vi "5.0.2_HL_Restriction.vi"(6 "Data in":T1, 8 "error in (no error)":errorcluster, 9 "AllControls In":T2, 10 "?":T3, 11 "Message Queue out":T4) -> (0 "error out":errorcluster, 1 "Flow":string, 2 "Data":T3, 3 "Message Queue Out":T4, 4 "Data out":T1)   [LabVIEW 2017]
uses:
  Depends/AMC/subVIs/TypeDefs/amc_Message Queue.ctl
  Depends/AMC/subVIs/TypeDefs/amc_Message.ctl
  Depends/Tools/Keyed Array/Tools_KeyedArray KeyedArray.ctl
  Ctrls/Data.ctl
  Ctrls/AllControls.ctl
  Ctrls/CSV_Data.ctl
  DIPC 692 Daemon API/typdef/get_parameter.ctl
  DIPC 692 Daemon API/typdef/task_detect_test_point.ctl
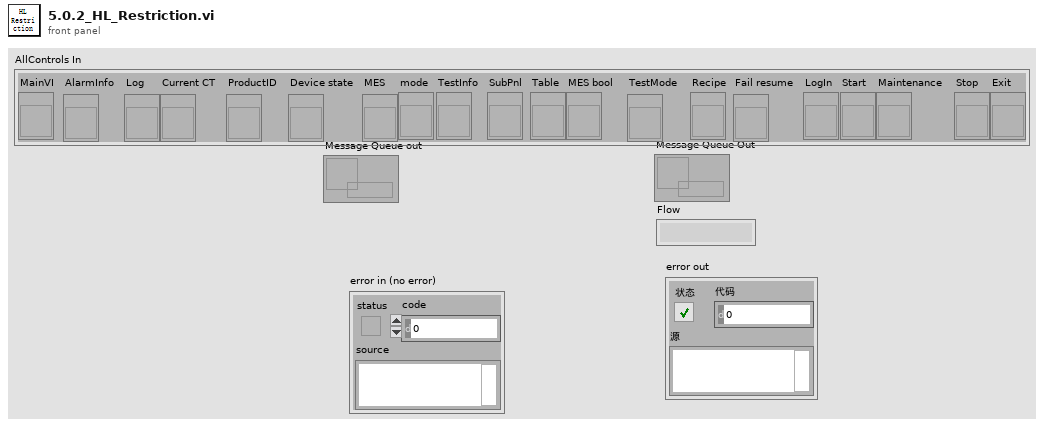
[diagram p1: front panel]
types:
  T1 = typedef "CSV_Data.ctl" = cluster{"Initialisation":cluster{"LMT - Connect UUT (con COM)":string, "LMT - Software Version (rrel)":string, "LMT - Write SKU file (wskuc)":string, "LMT - SKU file name":string, "Connect UUT DDM":string, "Read DDM EOL Timestamp - Mode":string, "Read DDM EOL Timestamp - Timestamp":string, "Read DDM EOL Timestamp - Rig ID":string, "Read DDM EOL Timestamp - Passmark ID":string, "Read DDM EOL Timestamp - Passmark Rev":string, "Software Version before flashing":string, "Read Hardware Serial":string, "UUT DDM SN":string, "Compare DDM SN with MES SN":string, "Backup PCBA Calibration EEPROM Response - CAL":string, "Flash Firmware Version":string, "Check SW Version":string, "Read DDM SW Version after flashing":string, "Set SKU Config":string, "Ready Status":string, "Set Device Mode to EOL":string, "DDM Parameter - Voltage":string, "DDM Parameter - Current":string, "DDM Parameter - Power":string, "DDM Parameter - Speed":string, "DDM Parameter - Pressure":string, "Tester Parameter - Voltage":string, "Tester Parameter - Current":string, "Tester Parameter - Power":string, "Tester Parameter - Ambient Pressure":string, "Tester Parameter - Ambient Temperature":string, "Calculated Parameter - DDM Pressure Corrected":string, "Calculated Parameter - DDM Real Power":string, "Calculated Parameter - Delta V":string}, "BEMF_Calibration":cluster{"Calibration Result - eol_cold_bemf_temp":string, "DDM Ambient Temp":string, "Restriction Plate Diameter":string, "Calibration Result - eol_bemf_mp_cold_coef_a":string, "Calibration Result - eol_bemf_mp_cold_coef_b":string, "Calibration Result - eol_bemf_mp_cold_coef_c":string, "Calibration Result - eol_bemf_lsi_cold_ref_coeffs":string, "Get - Calibration Result - eol_bemf_lsi_speed":string, "Get - Calibration Result - eol_bemf_lsi_integral_0":string, "Calibration Result - eol_bemf_lsi_integral_1":string, "Get - Calibration Result - eol_bemf_lsi_integral_2":string, "Get - Calibration Result - eol_cold_bemf":string, "Get - Calibration Result - eol_cold_bemf_fisf":string, "Finalise Calibration":string, "Compare -Calibration Result - eol_cold_bemf":string, "Compare -Calibration Result - eol_cold_bemf_fisf":string}, "ECO":cluster{"Reset Power Tune":string, "Reset BEMF FISF Calibration":string, "Restriction Plate Diameter":string, "ECO - Stabilisation Time":string, "ECO - DDM Parameter - Voltage":string, "ECO - DDM Parameter - Current":string, "ECO - DDM Parameter - Power":string, "ECO - DDM Parameter - Measured Power":string, "ECO - DDM Parameter - Speed":string, "ECO - DDM Parameter - Pressure":string, "ECO - Tester Parameter - Voltage":string, "ECO - Tester Parameter - Current":string, "ECO - Tester Parameter - Power":string, "ECO - Tester Parameter - Ambient Pressure":string, "ECO - Tester Parameter - Ambient Temperature":string, "ECO - Tester Parameter - Ambient Humidity":string, "ECO - Calculated Parameter - DDM Pressure Corrected":string, "ECO - Calculated Parameter - DDM Real Power":string, "ECO - Calculated Parameter - Delta V":string, "ECO - Calculated Parameter - Flowrate":string, "ECO - Calculated Parameter - Airwatt":string, "ECO - Formula":string, "PT ECO - Power Tune Mode Status":string}, "BOOST":cluster{"Restriction Plate Diameter":string, "BOOST - Stabilisation Time":string, "BOOST - DDM Parameter - Voltage":string, "BOOST - DDM Parameter - Current":string, "BOOST - DDM Parameter - Power":string, "BOOST - DDM Parameter - Measured Power":string, "BOOST - DDM Parameter - Speed":string, "BOOST - DDM Parameter - Pressure":string, "BOOST - Tester Parameter - Voltage":string, "BOOST - Tester Parameter - Current":string, "BOOST - Tester Parameter - Power":string, "BOOST - Tester Parameter - Ambient Pressure":string, "BOOST - Tester Parameter - Ambient Temperature":string, "BOOST - Tester Parameter - Ambient Humidity":string, "BOOST - Calculated Parameter - DDM Pressure Corrected":string, "BOOST - Calculated Parameter - DDM Real Power":string, "BOOST - Calculated Parameter - Delta V":string, "BOOST - Calculated Parameter - Flowrate":string, "BOOST - Calculated Parameter - Airwatt":string, "BOOST - Get AM Presence":string, "Air Muscle Turn Off Status":string, "BOOST - Air Muscle Calculated Parameter - Airwatt B":string, "BOOST - Air Muscle Calculate Airwatt Delta":string, "PT BOOST - Power Tune Mode Status":string, "Finalise Calibration":string, "ECO - Get AW Calibration value":string, "BOOST - Get AW Calibration value":string}, "MAX":cluster{"Restriction Plate Diameter":string, "MAX - Stabilisation Time":string, "Get Average Delta Tmag (LSIdelta_FISFdelta_LSItmag_FISFtmag_IIRtmag)":string, "Get Average Delta Tmag FISF":string, "MAX - DDM Parameter - Voltage":string, "MAX - DDM Parameter - Current":string, "MAX - DDM Parameter - Power":string, "MAX - DDM Parameter - Measured Power":string, "MAX - DDM Parameter - Speed":string, "MAX - DDM Parameter - Pressure":string, "MAX - Tester Parameter - Voltage":string, "MAX - Tester Parameter - Current":string, "MAX - Tester Parameter - Power":string, "MAX - Tester Parameter - Ambient Pressure":string, "MAX - Tester Parameter - Ambient Temperature":string, "MAX - Tester Parameter - Ambient Humidity":string, "MAX - Calculated Parameter - DDM Pressure Corrected":string, "MAX - Calculated Parameter - DDM Real Power":string, "MAX - Calculated Parameter - Delta V":string, "MAX - Calculated Parameter - Flowrate":string, "MAX - Calculated Parameter - Airwatt":string, "MAX_FISF_Check_Average_Delta_Tmag":string, "MAX - FISF - BEMF Finetune Result":string, "MAX tune - Delta P1":string, "MAX tune - Calculated Parameter - Airwatt":string, "Calculate Delta Airwatts - MAX finetune - Delta P2":string, "MAX finetune - DDM Parameter - Voltage":string, "MAX finetune - DDM Parameter - Current":string, "MAX finetune - DDM Parameter - Power":string, "MAX finetune - DDM Parameter - Measured Power":string, "MAX finetune - DDM Parameter - Speed":string, "MAX finetune - DDM Parameter - Pressure":string, "MAX finetune - Tester Parameter - Voltage":string, "MAX finetune - Tester Parameter - Current":string, "MAX finetune - Tester Parameter - Power":string, "MAX finetune - Tester Parameter - Ambient Pressure":string, "MAX finetune - Tester Parameter - Ambient Temperature":string, "MAX finetune - Tester Parameter - Ambient Humidity":string, "MAX finetune - Calculated Parameter - DDM Pressure Corrected":string, "MAX finetune - Calculated Parameter - DDM Real Power":string, "MAX finetune - Calculated Parameter - Delta V":string, "MAX finetune - Calculated Parameter - Flowrate":string, "MAX finetune - Calculated Parameter - Airwatt":string, "Check Derate Result":string, "Delta Tmag FISF":string, "Get Hot BEMF Result":string, "Calculate delta Pressure":string, "Finalise Calibration":string, "Calculate & Check Delta BEMF":string, "Delta P Airwatts Value":string}, "LL":cluster{"DDM Ambient Temp":string, "Restriction Plate Diameter":string, "LL - DDM Parameter - Voltage":string, "LL - DDM Parameter - Current":string, "LL - DDM Parameter - Power":string, "LL - DDM Parameter - Measured Power":string, "LL - DDM Parameter - Speed":string, "LL - DDM Parameter - Pressure":string, "LL - Tester Parameter - Voltage":string, "LL - Tester Parameter - Current":string, "LL - Tester Parameter - Power":string, "LL - DDM Real Power":string, "LL - Calibrate Task Detect LL":string}, "HL":cluster{"HL - DDM Parameter - Voltage":string, "HL - DDM Parameter - Current":string, "HL - DDM Parameter - Power":string, "HL - DDM Parameter - Measured Power":string, "HL - DDM Parameter - Speed":string, "HL - DDM Parameter - Pressure":string, "HL - Tester Parameter - Voltage":string, "HL - Tester Parameter - Current":string, "HL - Tester Parameter - Power":string, "HL - DDM Real Power":string, "HL - Calibrate Task Detect HL":string}, "LH":cluster{"Restriction Plate Diameter":string, "LH - DDM Parameter - Voltage":string, "LH - DDM Parameter - Current":string, "LH - DDM Parameter - Power":string, "LH - DDM Parameter - Measured Power":string, "LH - DDM Parameter - Speed":string, "LH - DDM Parameter - Pressure":string, "LH - Tester Parameter - Voltage":string, "LH - Tester Parameter - Current":string, "LH - Tester Parameter - Power":string, "LH - DDM Real Power":string, "LH - Calibrate Task Detect LH":string}, "HH":cluster{"HH - DDM Parameter - Voltage":string, "HH - DDM Parameter - Current":string, "HH - DDM Parameter - Power":string, "HH - DDM Parameter - Measured Power":string, "HH - DDM Parameter - Speed":string, "HH - DDM Parameter - Pressure":string, "HH - Tester Parameter - Voltage":string, "HH - Tester Parameter - Current":string, "HH - Tester Parameter - Power":string, "HH - DDM Real Power":string, "HH - Calibrate Task Detect HH":string}, "Inlet Blockage Calibration":cluster{"Inlet Blockage Calibration - DDM Parameter - Voltage":string, "Inlet Blockage Calibration - DDM Parameter - Current":string, "Inlet Blockage Calibration - DDM Parameter - Power":string, "Inlet Blockage Calibration - DDM Parameter - Measured Power":string, "Inlet Blockage Calibration - DDM Parameter - Speed":string, "Inlet Blockage Calibration - DDM Parameter - Pressure":string, "Inlet Blockage Calibration - Tester Parameter - Voltage":string, "Inlet Blockage Calibration - Tester Parameter - Current":string, "Inlet Blockage Calibration - Tester Parameter - Power":string, "Inlet Blockage Calibration - DDM Real Power":string, "Calibration Inlet Blockage_E":string, "Finalise Calibration":string, "Get Task Detect LL":string, "Get Task Detect HL":string, "Get Task Detect LH":string, "Get Task Detect HH":string, "Calibration Inlet Blockage":string, "Calibration eol cold bemf temp":string}, "GOOD":cluster{"GOOD UNIT - Clear EEPROM Error Log":string, "GOOD UNIT - Write Product Timestamp - Mode":string, "GOOD UNIT - Write Product Timestamp - Timestamp":string, "GOOD UNIT - Write Product Timestamp - Rig ID":string, "GOOD UNIT - Write Product Timestamp - Passmark ID":string, "GOOD UNIT - Write Product Timestamp - Passmark Rev":string, "GOOD UNIT - Set Device Mode to PROD":string, "GOOD UNIT - Backup PCBA Calibration EEPROM Response":string, "GOOD UNIT - Check Security Bit":string, "GOOD UNIT - Set Calibration Lock":string, "GOOD UNIT - Get_Calibration_Lock":string, "GOOD UNIT - Disconnect UUT":string}, "NG":cluster{"NG UNIT - Read NVM Error":string, "NG UNIT - Set Device Mode to FCT":string, "NG UNIT - Backup PCBA Calibration EEPROM Response - CAL":string, "NG UNIT - Backup PCBA Calibration EEPROM Response - ERROR":string, "NG UNIT - Backup PCBA Calibration EEPROM Response - USAGE":string, "NG UNIT - Disconnect UUT":string}, "SN":string, "Table":string[][], "Count":cluster{"Total":i32, "OK":i32, "NG":i32, "Yield":dbl}, "Start Time":timestamp, "daemon reference":refnum<k5>, "CT":dbl, "Config":string[][], "OK/NG":bool, "Station ID":string, "MES DDM SN":string, "MES PCBA SN":string, "Retest":string, "UID":string, "Initialisation_Status":cluster{"LMT - Connect UUT (con COM)":string, "LMT - Software Version (rrel)":string, "LMT - Write SKU file (wskuc)":string, "LMT - SKU file name":string, "Connect UUT DDM":string, "Read DDM EOL Timestamp - Mode":string, "Read DDM EOL Timestamp - Timestamp":string, "Read DDM EOL Timestamp - Rig ID":string, "Read DDM EOL Timestamp - Passmark ID":string, "Read DDM EOL Timestamp - Passmark Rev":string, "Software Version before flashing":string, "Read Hardware Serial":string, "UUT DDM SN":string, "Compare DDM SN with MES SN":string, "Backup PCBA Calibration EEPROM Response - CAL":string, "Flash Firmware Version":string, "Check SW Version":string, "Read DDM SW Version after flashing":string, "Set SKU Config":string, "Ready Status":string, "Set Device Mode to EOL":string, "DDM Parameter - Voltage":string, "DDM Parameter - Current":string, "DDM Parameter - Power":string, "DDM Parameter - Speed":string, "DDM Parameter - Pressure":string, "Tester Parameter - Voltage":string, "Tester Parameter - Current":string, "Tester Parameter - Power":string, "Tester Parameter - Ambient Pressure":string, "Tester Parameter - Ambient Temperature":string, "Calculated Parameter - DDM Pressure Corrected":string, "Calculated Parameter - DDM Real Power":string, "Calculated Parameter - Delta V":string}, "BEMF_Calibration_Status":cluster{"Calibration Result - eol_cold_bemf_temp":string, "DDM Ambient Temp":string, "Restriction Plate Diameter":string, "Calibration Result - eol_bemf_mp_cold_coef_a":string, "Calibration Result - eol_bemf_mp_cold_coef_b":string, "Calibration Result - eol_bemf_mp_cold_coef_c":string, "Calibration Result - eol_bemf_lsi_cold_ref_coeffs":string, "Get - Calibration Result - eol_bemf_lsi_speed":string, "Get - Calibration Result - eol_bemf_lsi_integral_0":string, "Calibration Result - eol_bemf_lsi_integral_1":string, "Get - Calibration Result - eol_bemf_lsi_integral_2":string, "Get - Calibration Result - eol_cold_bemf":string, "Get - Calibration Result - eol_cold_bemf_fisf":string, "Finalise Calibration":string, "Compare -Calibration Result - eol_cold_bemf":string, "Compare -Calibration Result - eol_cold_bemf_fisf":string}, "ECO_Status":cluster{"Reset Power Tune":string, "Reset BEMF FISF Calibration":string, "Restriction Plate Diameter":string, "ECO - Stabilisation Time":string, "ECO - DDM Parameter - Voltage":string, "ECO - DDM Parameter - Current":string, "ECO - DDM Parameter - Power":string, "ECO - DDM Parameter - Measured Power":string, "ECO - DDM Parameter - Speed":string, "ECO - DDM Parameter - Pressure":string, "ECO - Tester Parameter - Voltage":string, "ECO - Tester Parameter - Current":string, "ECO - Tester Parameter - Power":string, "ECO - Tester Parameter - Ambient Pressure":string, "ECO - Tester Parameter - Ambient Temperature":string, "ECO - Tester Parameter - Ambient Humidity":string, "ECO - Calculated Parameter - DDM Pressure Corrected":string, "ECO - Calculated Parameter - DDM Real Power":string, "ECO - Calculated Parameter - Delta V":string, "ECO - Calculated Parameter - Flowrate":string, "ECO - Calculated Parameter - Airwatt":string, "ECO - Formula":string, "PT ECO - Power Tune Mode Status":string}, "BOOST_Status":cluster{"Restriction Plate Diameter":string, "BOOST - Stabilisation Time":string, "BOOST - DDM Parameter - Voltage":string, "BOOST - DDM Parameter - Current":string, "BOOST - DDM Parameter - Power":string, "BOOST - DDM Parameter - Measured Power":string, "BOOST - DDM Parameter - Speed":string, "BOOST - DDM Parameter - Pressure":string, "BOOST - Tester Parameter - Voltage":string, "BOOST - Tester Parameter - Current":string, "BOOST - Tester Parameter - Power":string, "BOOST - Tester Parameter - Ambient Pressure":string, "BOOST - Tester Parameter - Ambient Temperature":string, "BOOST - Tester Parameter - Ambient Humidity":string, "BOOST - Calculated Parameter - DDM Pressure Corrected":string, "BOOST - Calculated Parameter - DDM Real Power":string, "BOOST - Calculated Parameter - Delta V":string, "BOOST - Calculated Parameter - Flowrate":string, "BOOST - Calculated Parameter - Airwatt":string, "BOOST - Get AM Presence":string, "Air Muscle Turn Off Status":string, "BOOST - Air Muscle Calculated Parameter - Airwatt B":string, "BOOST - Air Muscle Calculate Airwatt Delta":string, "PT BOOST - Power Tune Mode Status":string, "Finalise Calibration":string, "ECO - Get AW Calibration value":string, "BOOST - Get AW Calibration value":string}, "MAX_Status":cluster{"Restriction Plate Diameter":string, "MAX - Stabilisation Time":string, "Get Average Delta Tmag (LSIdelta_FISFdelta_LSItmag_FISFtmag_IIRtmag)":string, "Get Average Delta Tmag FISF":string, "MAX - DDM Parameter - Voltage":string, "MAX - DDM Parameter - Current":string, "MAX - DDM Parameter - Power":string, "MAX - DDM Parameter - Measured Power":string, "MAX - DDM Parameter - Speed":string, "MAX - DDM Parameter - Pressure":string, "MAX - Tester Parameter - Voltage":string, "MAX - Tester Parameter - Current":string, "MAX - Tester Parameter - Power":string, "MAX - Tester Parameter - Ambient Pressure":string, "MAX - Tester Parameter - Ambient Temperature":string, "MAX - Tester Parameter - Ambient Humidity":string, "MAX - Calculated Parameter - DDM Pressure Corrected":string, "MAX - Calculated Parameter - DDM Real Power":string, "MAX - Calculated Parameter - Delta V":string, "MAX - Calculated Parameter - Flowrate":string, "MAX - Calculated Parameter - Airwatt":string, "MAX_FISF_Check_Average_Delta_Tmag":string, "MAX - FISF - BEMF Finetune Result":string, "MAX tune - Delta P1":string, "MAX tune - Calculated Parameter - Airwatt":string, "Calculate Delta Airwatts - MAX finetune - Delta P2":string, "MAX finetune - DDM Parameter - Voltage":string, "MAX finetune - DDM Parameter - Current":string, "MAX finetune - DDM Parameter - Power":string, "MAX finetune - DDM Parameter - Measured Power":string, "MAX finetune - DDM Parameter - Speed":string, "MAX finetune - DDM Parameter - Pressure":string, "MAX finetune - Tester Parameter - Voltage":string, "MAX finetune - Tester Parameter - Current":string, "MAX finetune - Tester Parameter - Power":string, "MAX finetune - Tester Parameter - Ambient Pressure":string, "MAX finetune - Tester Parameter - Ambient Temperature":string, "MAX finetune - Tester Parameter - Ambient Humidity":string, "MAX finetune - Calculated Parameter - DDM Pressure Corrected":string, "MAX finetune - Calculated Parameter - DDM Real Power":string, "MAX finetune - Calculated Parameter - Delta V":string, "MAX finetune - Calculated Parameter - Flowrate":string, "MAX finetune - Calculated Parameter - Airwatt":string, "Check Derate Result":string, "Delta Tmag FISF":string, "Get Hot BEMF Result":string, "Calculate delta Pressure":string, "Finalise Calibration":string, "Calculate & Check Delta BEMF":string, "Delta P Airwatts Value":string}, "LL_Status":cluster{"DDM Ambient Temp":string, "Restriction Plate Diameter":string, "LL - DDM Parameter - Voltage":string, "LL - DDM Parameter - Current":string, "LL - DDM Parameter - Power":string, "LL - DDM Parameter - Measured Power":string, "LL - DDM Parameter - Speed":string, "LL - DDM Parameter - Pressure":string, "LL - Tester Parameter - Voltage":string, "LL - Tester Parameter - Current":string, "LL - Tester Parameter - Power":string, "LL - DDM Real Power":string, "LL - Calibrate Task Detect LL":string}, "HL_Status":cluster{"HL - DDM Parameter - Voltage":string, "HL - DDM Parameter - Current":string, "HL - DDM Parameter - Power":string, "HL - DDM Parameter - Measured Power":string, "HL - DDM Parameter - Speed":string, "HL - DDM Parameter - Pressure":string, "HL - Tester Parameter - Voltage":string, "HL - Tester Parameter - Current":string, "HL - Tester Parameter - Power":string, "HL - DDM Real Power":string, "HL - Calibrate Task Detect HL":string}, "LH_Status":cluster{"Restriction Plate Diameter":string, "LH - DDM Parameter - Voltage":string, "LH - DDM Parameter - Current":string, "LH - DDM Parameter - Power":string, "LH - DDM Parameter - Measured Power":string, "LH - DDM Parameter - Speed":string, "LH - DDM Parameter - Pressure":string, "LH - Tester Parameter - Voltage":string, "LH - Tester Parameter - Current":string, "LH - Tester Parameter - Power":string, "LH - DDM Real Power":string, "LH - Calibrate Task Detect LH":string}, "HH_Status":cluster{"HH - DDM Parameter - Voltage":string, "HH - DDM Parameter - Current":string, "HH - DDM Parameter - Power":string, "HH - DDM Parameter - Measured Power":string, "HH - DDM Parameter - Speed":string, "HH - DDM Parameter - Pressure":string, "HH - Tester Parameter - Voltage":string, "HH - Tester Parameter - Current":string, "HH - Tester Parameter - Power":string, "HH - DDM Real Power":string, "HH - Calibrate Task Detect HH":string}, "Inlet Blockage Calibration_Status":cluster{"Inlet Blockage Calibration - DDM Parameter - Voltage":string, "Inlet Blockage Calibration - DDM Parameter - Current":string, "Inlet Blockage Calibration - DDM Parameter - Power":string, "Inlet Blockage Calibration - DDM Parameter - Measured Power":string, "Inlet Blockage Calibration - DDM Parameter - Speed":string, "Inlet Blockage Calibration - DDM Parameter - Pressure":string, "Inlet Blockage Calibration - Tester Parameter - Voltage":string, "Inlet Blockage Calibration - Tester Parameter - Current":string, "Inlet Blockage Calibration - Tester Parameter - Power":string, "Inlet Blockage Calibration - DDM Real Power":string, "Calibration Inlet Blockage_E":string, "Finalise Calibration":string, "Get Task Detect LL":string, "Get Task Detect HL":string, "Get Task Detect LH":string, "Get Task Detect HH":string, "Calibration Inlet Blockage":string, "Calibration eol cold bemf temp":string}, "GOOD_Status":cluster{"GOOD UNIT - Clear EEPROM Error Log":string, "GOOD UNIT - Write Product Timestamp - Mode":string, "GOOD UNIT - Write Product Timestamp - Timestamp":string, "GOOD UNIT - Write Product Timestamp - Rig ID":string, "GOOD UNIT - Write Product Timestamp - Passmark ID":string, "GOOD UNIT - Write Product Timestamp - Passmark Rev":string, "GOOD UNIT - Set Device Mode to PROD":string, "GOOD UNIT - Backup PCBA Calibration EEPROM Response":string, "GOOD UNIT - Check Security Bit":string, "GOOD UNIT - Set Calibration Lock":string, "GOOD UNIT - Get_Calibration_Lock":string, "GOOD UNIT - Disconnect UUT":string}, "NG_Status":cluster{"NG UNIT - Read NVM Error":string, "NG UNIT - Set Device Mode to FCT":string, "NG UNIT - Backup PCBA Calibration EEPROM Response - CAL":string, "NG UNIT - Backup PCBA Calibration EEPROM Response - ERROR":string, "NG UNIT - Backup PCBA Calibration EEPROM Response - USAGE":string, "NG UNIT - Disconnect UUT":string}, "SKU":string, "Plate_Diameter":string, "Alarm":string}
  T2 = typedef "AllControls.ctl" = cluster{"MainVI":refnum<vi>, "AlarmInfo":refnum<vi>, "Log":refnum<vi>, "Current CT":refnum<vi>, "ProductID":refnum<vi>, "Device state":refnum<vi>, "MES":refnum<vi>, "mode":refnum<vi>, "TestInfo":refnum<vi>, "SubPnl":refnum<vi>, "Table":refnum<vi>, "MES bool":refnum<vi>, "TestMode":refnum<vi>, "Recipe":refnum<vi>, "Fail resume":refnum<vi>, "LogIn":refnum<vi>, "Start":refnum<vi>, "Maintenance":refnum<vi>, "Stop":refnum<vi>, "Exit":refnum<vi>}
  T3 = typedef "Data.ctl" = cluster{"Initialisation":cluster{"DDM_Parameter":dbl[], "DDM_Parameter_status":bool[], "Get_Tester_Parameter":dbl[], "Get_Tester_Parameter_status":bool[], "Cal_Tester_Parameter":dbl[], "Cal_Tester_Parameter_status":bool[], "sw_version_before_status":bool, "sw_version_after_status":bool, "Set_SKU_Config_With_LMT_status":bool, "FCT_timestamp_status":bool, "LMT_Connect_to_UUT_status":bool}, "BEMF_Calibration":cluster{"Read_ambient_temperature":dbl, "Calibration_Vaule":dbl[], "Calibration_Vaule _B":dbl[], "Calibration_Vaule_status":bool[], "Calibration_Vaule_B_status":bool[]}, "ECO":cluster{"DDM_Parameter":dbl[], "DDM_Parameter_status":bool[], "Get_Tester_Parameter":dbl[], "Get_Tester_Parameter_status":bool[], "Cal_Tester_Parameter":dbl[], "Cal_Tester_Parameter_status":bool[], "DDM_Parameter_after_power_tune":dbl[], "Get_Tester_Parameter_after_power_tune":dbl[], "Cal_Tester_Parameter_after_power_tune":dbl[], "Cal_Tester_Parameter_after_power_tune_status":bool[], "Delta_P":dbl}, "BOOST":cluster{"DDM_Parameter":dbl[], "DDM_Parameter_status":bool[], "Get_Tester_Parameter":dbl[], "Get_Tester_Parameter_status":bool[], "Cal_Tester_Parameter":dbl[], "Cal_Tester_Parameter_status":bool[], "DDM_Parameter_after_power_tune":dbl[], "Get_Tester_Parameter_after_power_tune":dbl[], "Cal_Tester_Parameter_after_power_tune":dbl[], "Cal_Tester_Parameter_after_power_tune_status":bool[], "airwatts_am_off":dbl, "AW_Delta_(AM_on_and_off)":dbl, "AW_Delta_(AM_on_and_off)_Status":bool, "Delta_P":dbl}, "MAX":cluster{"Average_Tmag_Data":cluster{"LSI Delta in degC":dbl, "FISF Delta in degc":dbl, "LSI Tmag in degC":dbl, "Fisf Tmag in degC":dbl, "IIR Tmag in degC":dbl}, "DDM_Parameter":dbl[], "DDM_Parameter_status":bool[], "Get_Tester_Parameter":dbl[], "Get_Tester_Parameter_status":bool[], "Cal_Tester_Parameter":dbl[], "BEMF_Finetune":cluster{"eol_bemf_mp_cold_coef_c":dbl, "eol_cold_bemf_fisf_offset":dbl}, "AW_Tune":cluster{"delta_P1":dbl, "delta_P_Setting":dbl}, "DDM_Parameter_after_Airwatts_Tune":dbl[], "Get_Tester_Parameter_after_Airwatts_Tune":dbl[], "Cal_Tester_Parameter_after_Airwatts_Tune":dbl[], "DDM_Parameter_after_Airwatts_Finetune":dbl[], "Get_Tester_Parameter_after_Airwatts_Finetune":dbl[], "Cal_Tester_Parameter_after_Airwatts_Finetune":dbl[], "AW_Finetune":cluster{"delta_P2":dbl, "delta_P_Setting":dbl}, "Delta_Tmag_after_tune":cluster{"LSI Delta in degC":dbl, "FISF Delta in degc":dbl, "LSI Tmag in degC":dbl, "Fisf Tmag in degC":dbl, "IIR Tmag in degC":dbl}, "Hot Bemf in mV":dbl, "DDM_Pressure":dbl, "Delta_Pressure":dbl, " Cold Bemf in mV":dbl, " delta Bemf":dbl, " delta p":dbl, "Delta_Pressure_status":bool, " delta Bemf_status":bool, "LSI Delta in degC_status":bool, "FISF Delta in degc_status":bool, "Max_check_derate_status_status":bool, "Average_All_data":dbl[][], "Average_Tmag_Data_status":bool[], "Average_Tmag_Data_after_tune_status":bool[], "Cal_Tester_Parameter_status":bool[], "Cal_Tester_Parameter_status_after_Airwatts_Tune":bool[], "Cal_Tester_Parameter_status_after_Airwatts_FineTune":bool[]}, "Task_Detect_Calib":cluster{"LL":cluster{"DDM_Parameter":dbl[], "DDM_Parameter_status":bool[], "Get_Tester_Parameter":dbl[], "Get_Tester_Parameter_status":bool[], "Set_task_detect_A":dbl, "Set_task_detect_A_Status":bool}, "HL":cluster{"DDM_Parameter":dbl[], "DDM_Parameter_status":bool[], "Get_Tester_Parameter":dbl[], "Get_Tester_Parameter_status":bool[], "Set_task_detect_B":dbl, "Set_task_detect_B_Status":bool}, "LH":cluster{"DDM_Parameter":dbl[], "DDM_Parameter_status":bool[], "Get_Tester_Parameter":dbl[], "Get_Tester_Parameter_status":bool[], "Set_task_detect_C":dbl, "Set_task_detect_C_Status":bool}, "HH":cluster{"DDM_Parameter":dbl[], "DDM_Parameter_status":bool[], "Get_Tester_Parameter":dbl[], "Get_Tester_Parameter_status":bool[], "Set_task_detect_D":dbl, "Read_and_check_calibration_Status":bool[], "Set_task_detect_D_Status":bool}, "Get_eol_inlet_blockage_E":dbl, "Calib_vaule":cluster{"Get_task_detect_LL":dbl, "Get_task_detect_HL":dbl, "Get_task_detect_LH":dbl, "Get_task_detect_HH":dbl, "eol_inlet_blockage":dbl, "eol_code_bemf_temp":dbl}, "calibrated temp":dbl, "Inlet_Blockage_Calibration":cluster{"DDM_Parameter":dbl[], "DDM_Parameter_status":bool[], "Get_Tester_Parameter":dbl[], "Get_Tester_Parameter_status":bool[]}, "Get_eol_inlet_blockage_E_Status":bool}, "good":cluster{"Write_Product_TS":cluster{"TIMESTAMP":i64, "RIG_ID":i64, "PASSMARK_ID":i64, "PASSMARK_REV":i64}, "Read_Product_TS":cluster{"TIMESTAMP":i64, "RIG_ID":i64, "PASSMARK_ID":i64, "PASSMARK_REV":i64}, "Good_Check_Secuity_Bit_Stauts":bool}}
  T4 = typedef "amc_Message Queue.ctl" = refnum<queue>
  T5 = typedef "HD Config.ctl" = cluster{" PC":cluster{"PC Address":u8[], "PC Port":i32}, "FCO":cluster{"COM":refnum<visa-resource-name>, "Baudrate":u32}, "DC Power ":cluster{"COM":refnum<visa-resource-name>, "Baudrate":u32}, "PW3336":cluster{"COM":refnum<visa-resource-name>, "Baudrate":u32}, "Lefoo":cluster{"COM":refnum<visa-resource-name>, "Baudrate":u32}, "AI Model":cluster{"COM":refnum<visa-resource-name>, "Baudrate":u32}, "DIPC":cluster{"COM":refnum<visa-resource-name>}, "RFID":cluster{"IP Address":string, "Port":u16, "Retry":u16}, "Motor":cluster{"COM":refnum<visa-resource-name>, "Baudrate":u32}, "Fail_resume_mode":bool, "GRR":bool}
  T6 = typedef "get_parameter.ctl" = string
  T7 = typedef "task_detect_test_point.ctl" = enum16{"LL", "HL", "LH", "HH"}
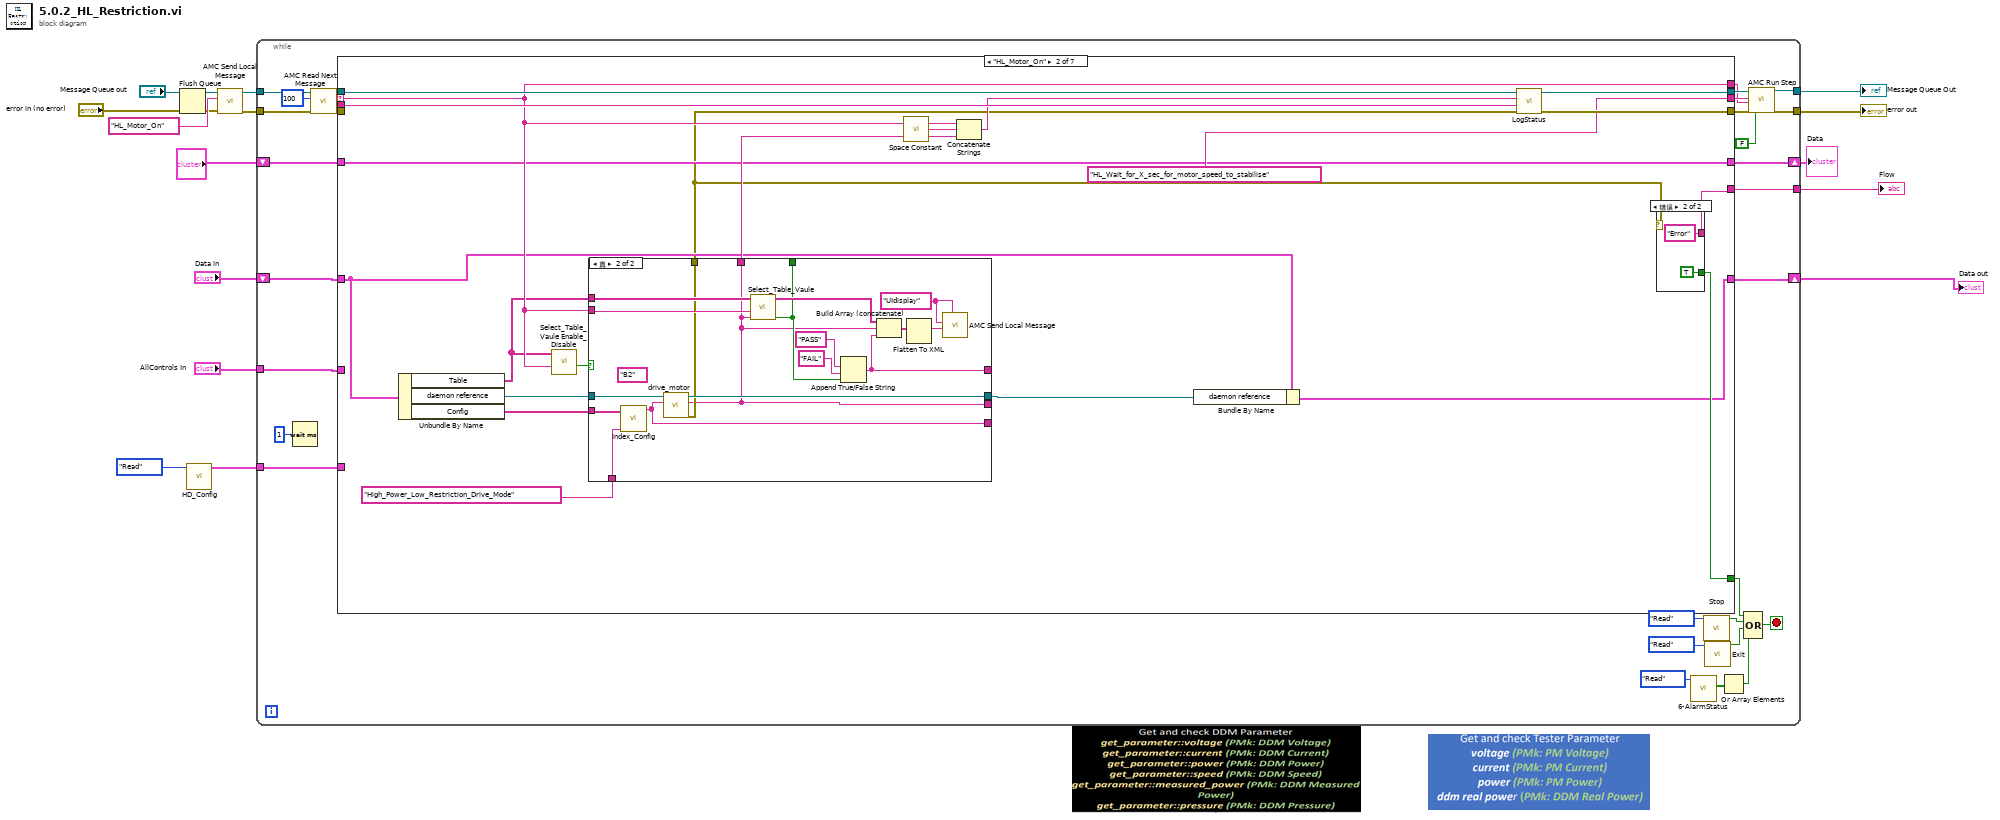
[diagram p0: block diagram]
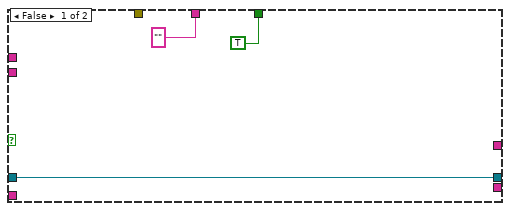
[diagram p4: hidden frame]
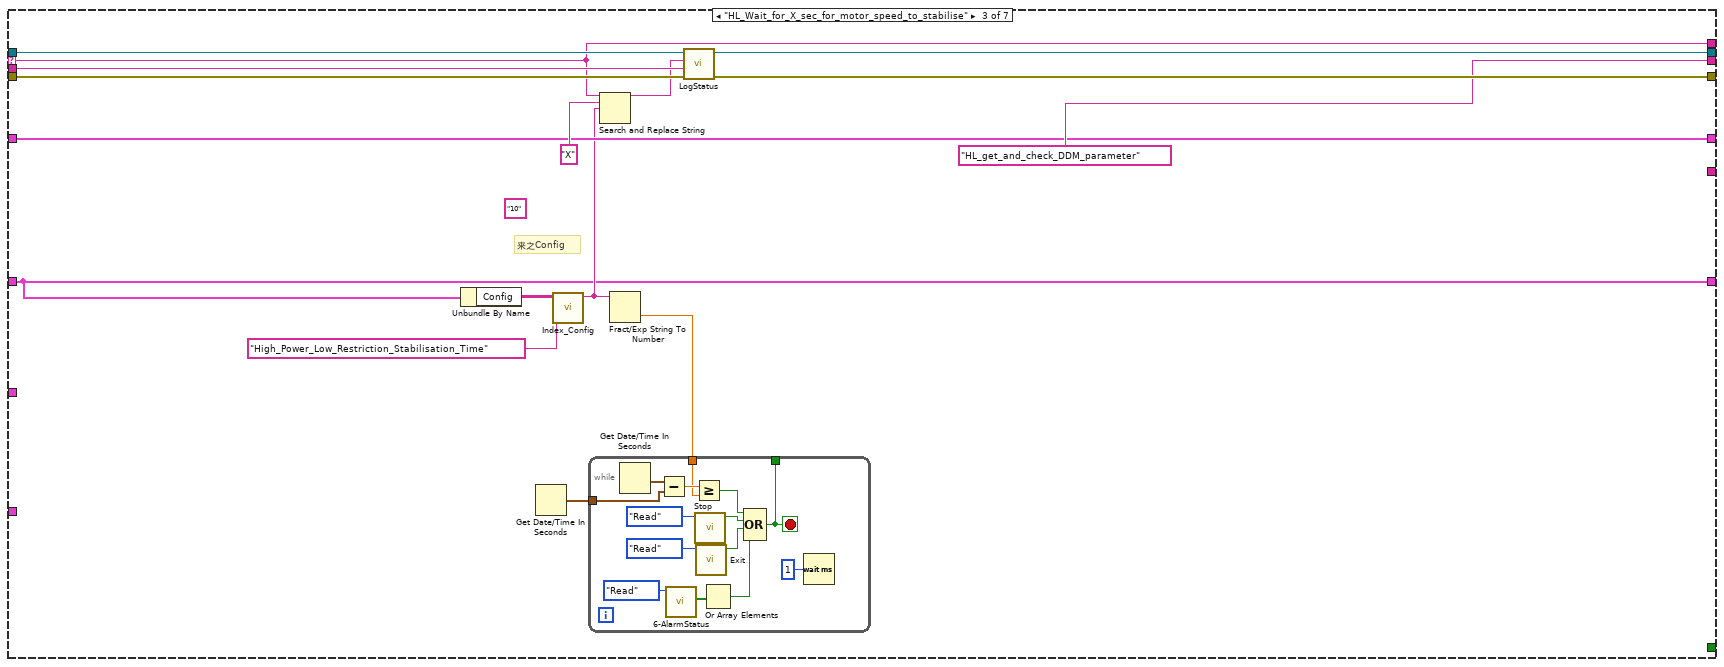
[diagram p5: hidden frame]
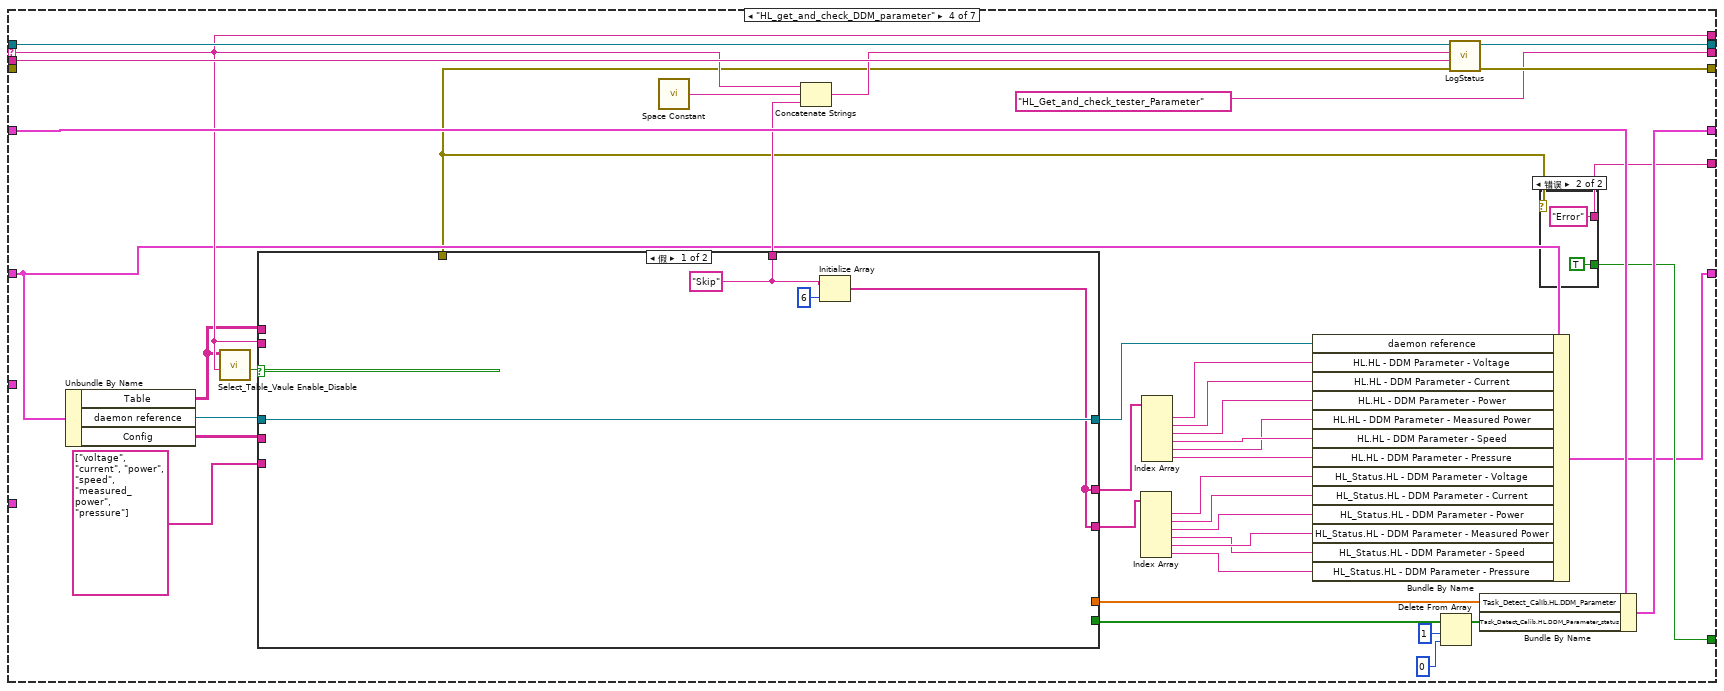
[diagram p6: hidden frame]
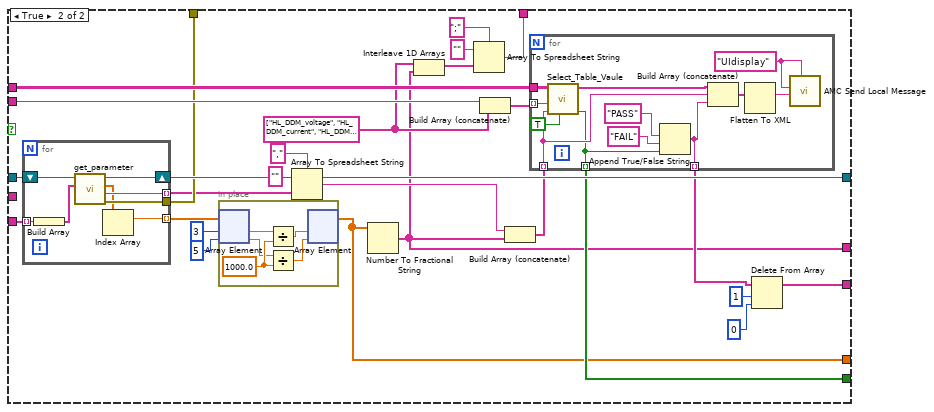
[diagram p8: hidden frame]
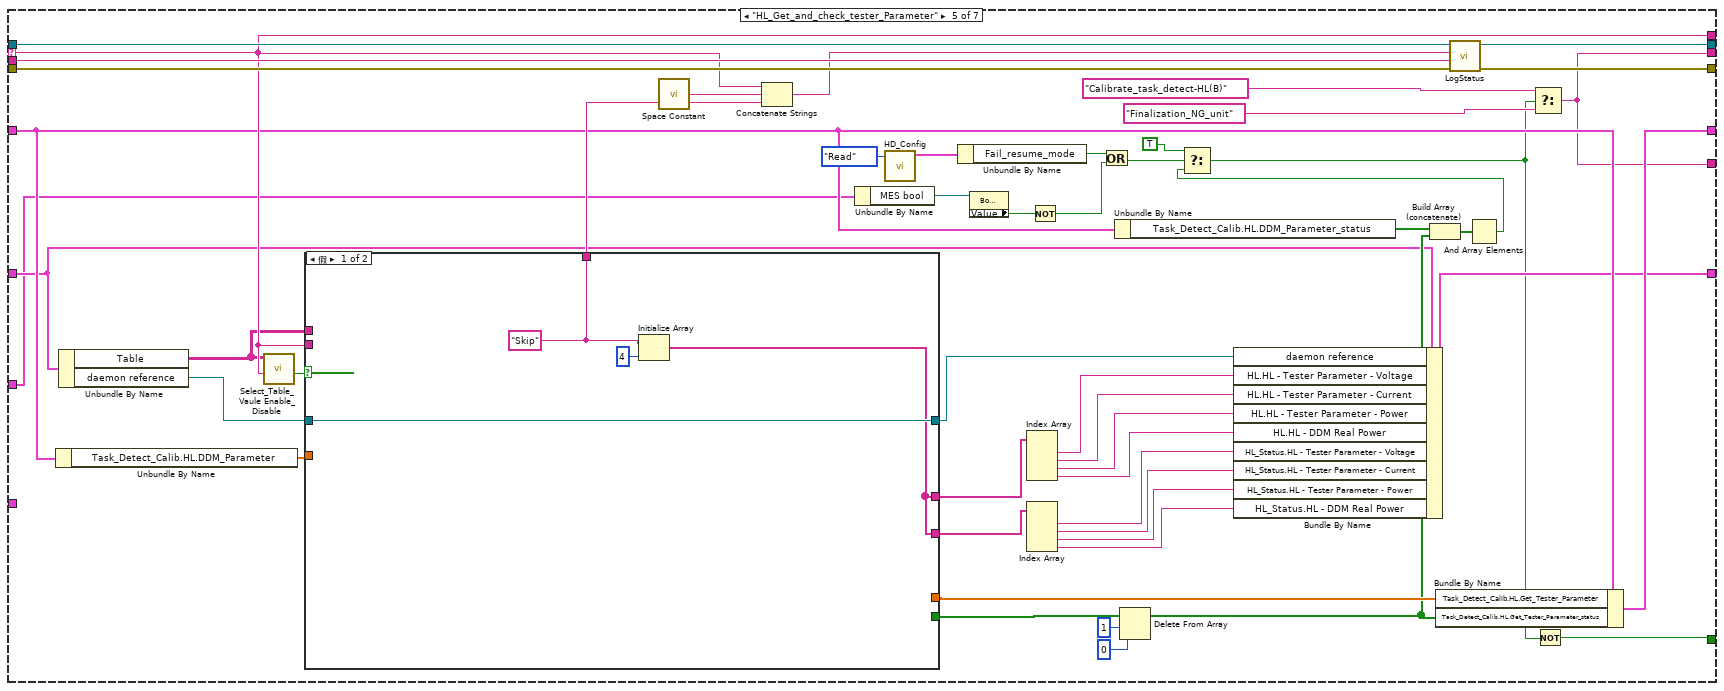
[diagram p9: hidden frame]
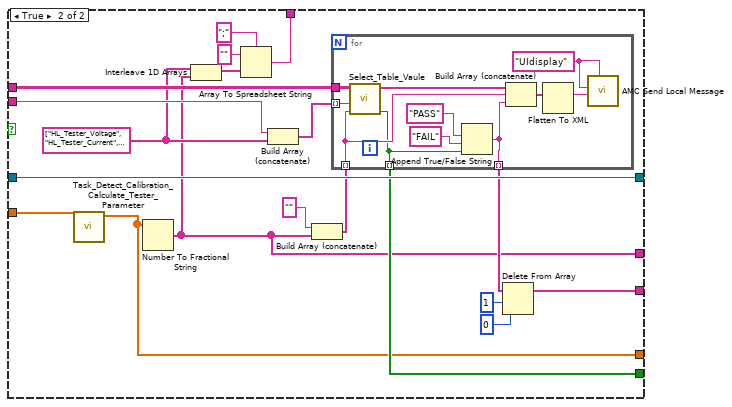
[diagram p10: hidden frame]
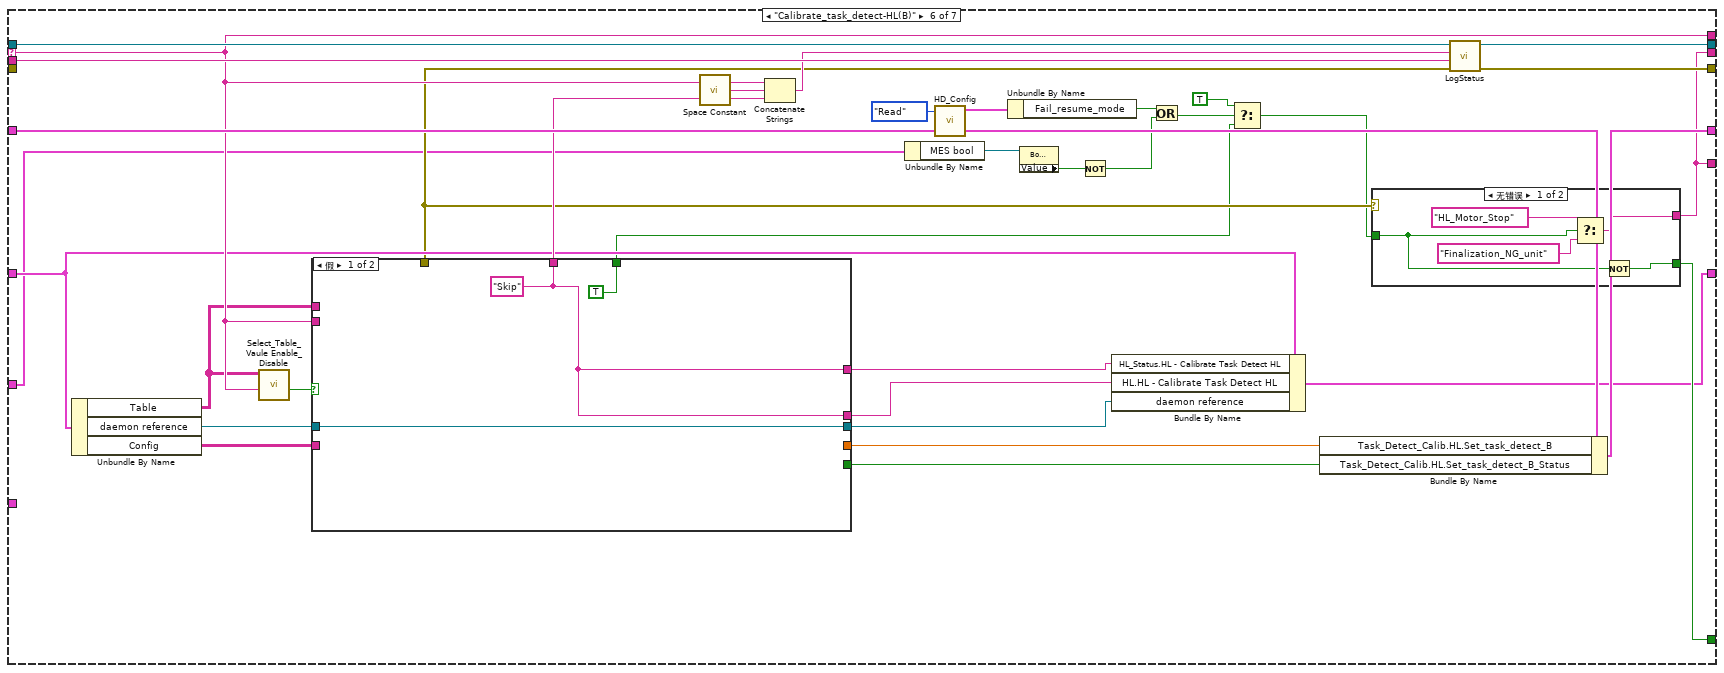
[diagram p11: hidden frame]
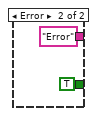
[diagram p12: hidden frame]
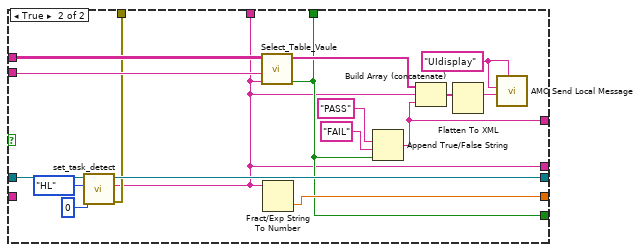
[diagram p13: hidden frame]
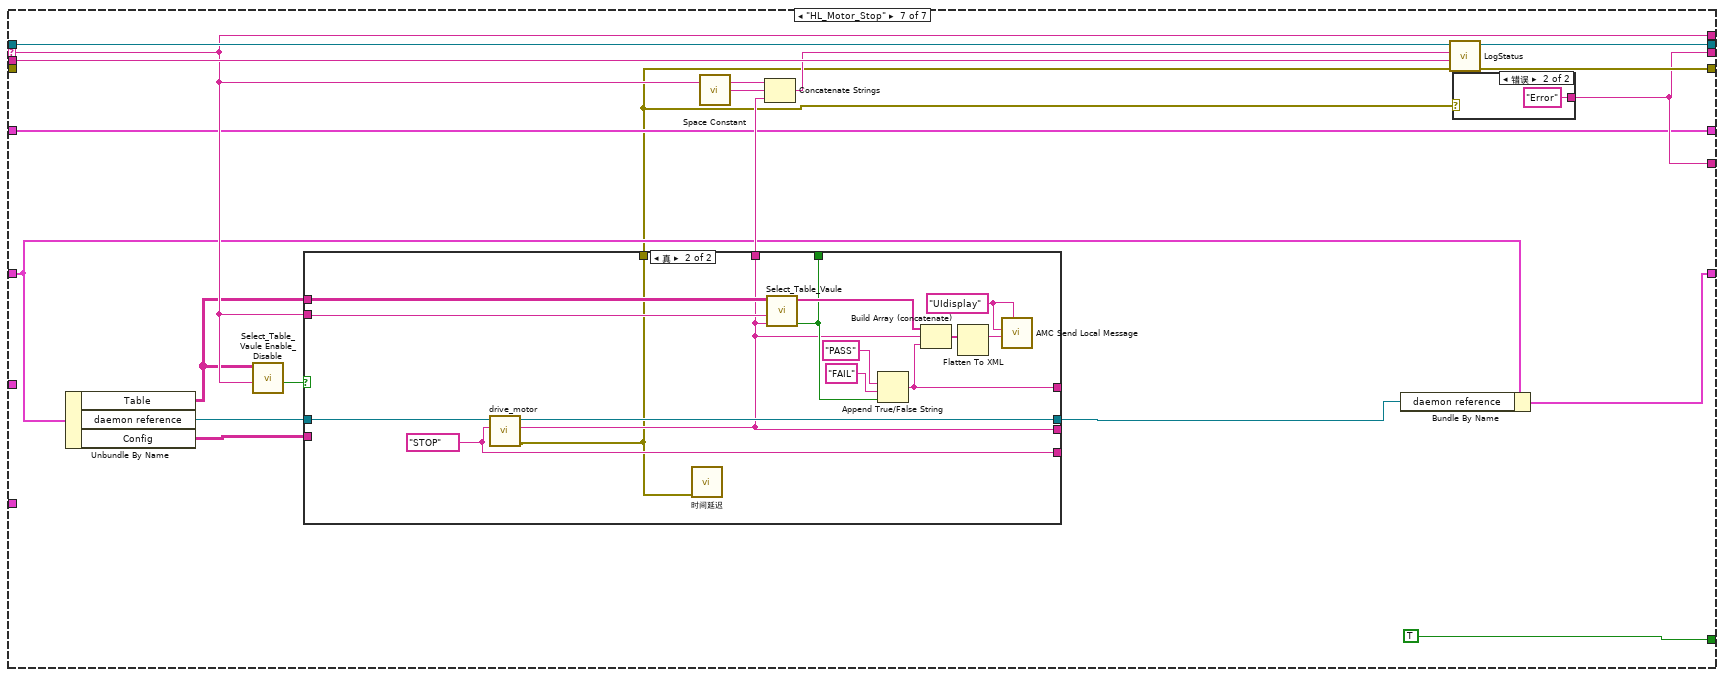
[diagram p14: hidden frame]
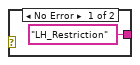
[diagram p15: hidden frame]
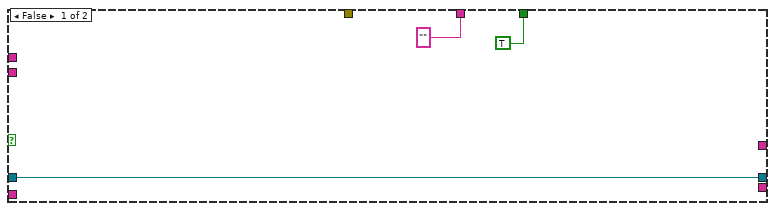
[diagram p16: hidden frame]
diagram:
  n1 = Flush Queue(queue="Message Queue out") -> (queue out=w4:T4)  [unwired: 1 in, 2 out]
  n2 = call "HD_Config.vi"("Step"=enum16{"Initial", "Write", "Read"}."Read") -> ("HD Config out"=w8:T5)  [unwired: 9 in, 1 out]
  n3 = call "AMC Send Local Message.vi"("error in (no error)"="error in (no error)", "Message Name"="HL_Motor_On", "Message Queue in"=w4) -> ("error out"=w13:errorcluster, "Message Queue out"=w14:T4)  [unwired: 7 in]
  n4 = while {
    tunnel: w14 -> [w47]
    tunnel: [w43] -> w6
    tunnel: w13 -> [w41]
    tunnel: [w38] -> w5
    shift-right: [w34] -> w10
    shift-left: "?" -> [w35]
    tunnel: w8 -> [w33]
    tunnel: [w29] -> w7
    shift-right: [w20] -> w1
    shift-left: "Data in" -> [w22]
    tunnel: "AllControls In" -> [w21]
    stop <- w23 stop-if-true
    n5 = Wait (ms)(milliseconds to wait=u32 1 ("等待时间（毫秒）")) -> ()  [unwired: 1 out]
    n6 = call "AMC Read Next Message.vi"("error in (no error)"=w41, "timeout (1ms)"=100, "Message Queue in"=w47) -> ("error out"=w40:errorcluster, "Message Value"=w31:string, "Message Name"=w45:string, "Message Queue out"=w46:T4)  [unwired: 1 in, 4 out]
    n7 = case shown="\"HL_Motor_On\"" w45 {
      selector: w45 -> [_ w64 w102 w153 w261 w327 w375]
      tunnel: w46 -> [w51 w71 w108 w162 w269 w337 w382]
      tunnel: [w51 w71 w108 w162 w269 w337 w382] -> w44
      tunnel: w40 -> [w50 _ w107 _ w268 _ _]
      tunnel: [w50 w70 w106 w161 w267 w336 w381] -> w39
      tunnel: [_ w58 _ w143 w253 w323 TRUE] -> w24
      tunnel: w35 -> [w49 w56 w100 w158 w256 w333 w369]
      tunnel: [w49 w56 w100 w157 w265 w332 w369] -> w34
      tunnel: w31 -> [_ w69 w105 w160 w266 w335 w380]
      tunnel: [_ w64 w102 w153 w261 w327 w375] -> w30
      tunnel: w33 -> [_ _ _ _ _ _ _]
      tunnel: [_ "HL_Wait_for_X_sec_for_motor_speed_to_stabilise" "HL_get_and_check_DDM_parameter" "HL_Get_and_check_tester_Parameter" w252 w317 w371] -> w32
      tunnel: [_ w59 _ w142 w252 w317 w371] -> w29
      tunnel: w22 -> [w48 w55 w94 w140 w244 w321 w368]
      tunnel: w21 -> [_ _ _ _ w232 w308 _]
      tunnel: [w48 w54 w94 w136 w241 w318 w367] -> w20
      frame "假", Default {
      }
      frame "HL_Motor_On" {
        n8 = Unbundle By Name(w55) -> ("Table"=w63:string[][], "daemon reference"=w68:refnum<k5>, "Config"=w61:string[][])
        n9 = call "Select_Table_Vaule Enable_Disable.vi"("Action"=w64, "Table"=w63) -> ("Enable"=w65:bool)  [unwired: 8 in, 1 out]
        n10 = case shown="真" w65 {
          tunnel: w68 -> [w75 w93]
          tunnel: [TRUE w83] -> _
          tunnel: [w75 w87] -> w52
          tunnel: ["" ("response") w79] -> w57
          tunnel: w64 -> [_ w86]
          tunnel: w63 -> [_ w85]
          tunnel: w61 -> [_ w82]
          tunnel: "High_Power_Low_Restriction_Drive_Mode" -> [_ w81]
          tunnel: [_ w80] -> w53
          tunnel: [_ w79] -> _
          tunnel: [_ w78] -> _
          tunnel: [_ w77] -> _
          frame False {
          }
          frame True {
            (unwired) "B2" ("Power Mode")
            w92 = "UIdisplay" ("Process (\"\" - local)")
            n11 = call "Index_Config.vi"("Action"=w81, "config"=w82) -> ("data"=w77:string)  [unwired: 9 in]
            n12 = call "drive_motor.vi"("Power Mode"=w77, "daemon reference in"=w93) -> ("error out"=w80:errorcluster, "response"=w79:string, "daemon reference out"=w87:refnum<k5>)  [unwired: 6 in, 1 out]
            n13 = call "Select_Table_Vaule.vi"("Vaule"=w79, "Action"=w86, "Table"=w85) -> ("Result"=w83:bool, "vaule"=w84:string[])  [unwired: 7 in]
            n14 = Append True/False String(1:w83, 2:"FAIL" ("真字符串"), 3:"PASS" ("真字符串")) -> (0:w78:string)  [unwired: 1 in]
            n15 = Build Array (concatenate)(w84, w79, w78) -> (w91:string[])
            n16 = Flatten To XML(anything=w91) -> (xml string=w90:string)
            n17 = call "AMC Send Local Message.vi"("Process (\"\" - local)"=w92, "Message Value"=w90, "Message Name"=w92) -> ()  [unwired: 7 in, 2 out]
          }
        }
        n18 = call <vilib>:"Space Constant.vi"() -> ("String"=w67:string)
        n19 = Concatenate Strings(w64, w67, w57) -> (w66:string)
        n20 = Bundle By Name(cluster=w55, "daemon reference"=w52) -> (w54:T1)
        n21 = call "LogStatus.vi"("error in (no error)"=w53, "last message"=w69, "message"=w66) -> ("error  out"=w70:errorcluster)  [unwired: 8 in]
        n22 = case shown="错误" w53 {
          tunnel: [_ TRUE] -> w58
          tunnel: [_ "Error"] -> w59
          frame No Error {
          }
          frame Error {
          }
        }
      }
      frame "HL_Wait_for_X_sec_for_motor_speed_to_stabilise" {
        (unwired) "10" ("替换字符串(\"\")")
        # "来之Config"
        n23 = Unbundle By Name(w94) -> ("Config"=w99:string[][])
        n24 = Get Date/Time In Seconds() -> (seconds since 1Jan1904=w96:timestamp)
        n25 = call "Index_Config.vi"("Action"="High_Power_Low_Restriction_Stabilisation_Time" ("替换字符串(\"\")"), "config"=w99) -> ("data"=w97:string)  [unwired: 9 in]
        n26 = Search and Replace String(input string=w102, search string="X" ("搜索字符串"), replace string=w97) -> (result string=w103:string)  [unwired: 5 in, 3 out]
        n27 = Fract/Exp String To Number(string=w97) -> (number=w95:dbl)  [unwired: 3 in, 1 out]
        n28 = while {
          tunnel: w96 -> [w115]
          tunnel: w95 -> [w112]
          tunnel: [w111] -> _
          stop <- w111 stop-if-true
          n29 = Get Date/Time In Seconds() -> (seconds since 1Jan1904=w116:timestamp)
          n30 = Subtract(x=w116, y=w115) -> (x-y=w114:dbl)
          n31 = call "6-AlarmStatus.vi"("Step"=enum16{"Initial", "Write", "Read"}."Read") -> ("AlarmValue Out"=w119:bool[])  [unwired: 9 in, 1 out]
          n32 = Greater Or Equal?(x=w114, y=w112) -> (x >= y?=w113:bool)
          n33 = call "Stop.vi"("Step"=enum16{"Initial", "Write", "Read"}."Read") -> ("Stop Out"=w117:bool)  [unwired: 9 in, 1 out]
          n34 = call "Exit.vi"("Step"=enum16{"Initial", "Write", "Read"}."Read" ("step")) -> ("Exit Out"=w121:bool)  [unwired: 9 in, 1 out]
          n35 = Or Array Elements(Boolean array=w119) -> (logical OR=w118:bool)
          n36 = Compound Arithmetic op=OR(w113, w117, w121, w118) -> (w111:bool)
          n37 = Wait (ms)(milliseconds to wait=u32 1 ("等待时间（毫秒）")) -> ()  [unwired: 1 out]
        }
        n38 = call "LogStatus.vi"("error in (no error)"=w107, "last message"=w105, "message"=w103) -> ("error  out"=w106:errorcluster)  [unwired: 8 in]
      }
      frame "HL_get_and_check_DDM_parameter" {
        n39 = Unbundle By Name(w140) -> ("Table"=w152:string[][], "daemon reference"=w159:refnum<k5>, "Config"=w150:string[][])
        n40 = call "Select_Table_Vaule Enable_Disable.vi"("Action"=w153, "Table"=w152) -> ("Enable"=w151:bool)  [unwired: 8 in, 1 out]
        n41 = case shown="假" w151 {
          tunnel: w159 -> [w168 w194]
          tunnel: [w168 w193] -> w137
          tunnel: [w167 w185] -> w154
          tunnel: w153 -> [_ w190]
          tunnel: w152 -> [_ w195]
          tunnel: w150 -> [_ _]
          tunnel: [_ w179] -> w148
          tunnel: [_ w192] -> w147
          tunnel: [_ w183] -> w138
          tunnel: T6[] ["voltage", "current", "power", "speed", "measured_power", "pressure"] ("Parameter") -> [_ w178]
          tunnel: [w166 w170] -> w139
          tunnel: [w166 w169] -> w129
          frame False {
            w167 = "Skip" ("software string")
            n42 = Initialize Array(w167, 6 ("维数大小")) -> (w166:string[])
          }
          frame True {
            w184 = string[] ["HL_DDM_voltage", "HL_DDM_current", "HL_DDM_power", "HL_DDM_speed", "HL_DDM_measured_power", "HL_DDM_pressure"]
            n43 = for {
              tunnel: [w201] -> w177 mode=indexing
              tunnel: [w200] -> w183
              tunnel: [w196] -> w180 mode=indexing
              tunnel: w178 -> [w198] mode=indexing
              shift-right: [w202] -> w193
              shift-left: w194 -> [w203]
              n44 = Build Array(w198) -> (w197:T6[])
              n45 = call "get_parameter.vi"("Parameter"=w197, "daemon reference in"=w203) -> ("error out"=w200:errorcluster, "response"=w201:string, "values"=w199:dbl[], "daemon reference out"=w202:refnum<k5>)  [unwired: 5 in, 1 out]
              n46 = Index Array(array=w199) -> (element=w196:dbl)  [unwired: 1 in]
            }
            n47 = in-place {
              w208 = 1000.0
              n48 = in-place-array #1(w180, 3, 5) -> (w207:dbl, w204:dbl)
              n49 = Divide(x=w207, y=w208) -> (x/y=w206:dbl)
              n50 = Divide(x=w204, y=w208) -> (x/y=w205:dbl)
              n51 = in-place-array #1(w206, w205) -> (w179:dbl[])  [unwired: 2 out]
            }
            n52 = Array To Spreadsheet String(delimiter (Tab)=",", array=w177, 3:"" ("format string")) -> (spreadsheet string=w174:string)
            n53 = Number To Fractional String(number=w179) -> (F-format string=w170:string[])  [unwired: 3 in]
            n54 = Interleave 1D Arrays(w184, w170) -> (w188:string[])
            n55 = Array To Spreadsheet String(delimiter (Tab)=";" ("格式字符串"), array=w188, 3:"" ("格式字符串")) -> (spreadsheet string=w185:string)
            n56 = Build Array (concatenate)(w190, w184) -> (w191:string[])
            n57 = Build Array (concatenate)(w174, w170) -> (w189:string[])
            n58 = for {
              tunnel: w195 -> [w215]
              tunnel: w189 -> [w213] mode=indexing
              tunnel: w191 -> [w212] mode=indexing
              tunnel: [w211] -> w192 mode=indexing
              tunnel: [w209] -> w171 mode=indexing
              w220 = "UIdisplay" ("Process (\"\" - local)")
              n59 = call "Select_Table_Vaule.vi"("Boolean"=TRUE, "Vaule"=w213, "Action"=w212, "Table"=w215) -> ("Result"=w211:bool, "vaule"=w214:string[])  [unwired: 6 in]
              n60 = Append True/False String(1:w211, 2:"FAIL" ("真字符串"), 3:"PASS" ("真字符串")) -> (0:w209:string)  [unwired: 1 in]
              n61 = Build Array (concatenate)(w214, w213, w209) -> (w219:string[])
              n62 = Flatten To XML(anything=w219) -> (xml string=w218:string)
              n63 = call "AMC Send Local Message.vi"("Process (\"\" - local)"=w220, "Message Value"=w218, "Message Name"=w220) -> ()  [unwired: 7 in, 2 out]
            }
            n64 = Delete From Array(array=w171, length=1 ("长度"), index=0 ("索引")) -> (array with subset deleted=w169:string[])  [unwired: 1 out]
          }
        }
        n65 = call <vilib>:"Space Constant.vi"() -> ("String"=w156:string)
        n66 = Concatenate Strings(w153, w156, w154) -> (w155:string)
        n67 = Index Array(array=w129) -> (element #1=w128:string, element #2=w127:string, element #3=w126:string, element #4=w124:string, element #5=w125:string, element #6=w123:string)  [unwired: 6 in]
        n68 = Index Array(array=w139) -> (element #1=w135:string, element #2=w134:string, element #3=w133:string, element #4=w132:string, element #5=w131:string, element #6=w130:string)  [unwired: 6 in]
        n69 = Bundle By Name(cluster=w140, "daemon reference"=w137, "HL.HL - DDM Parameter - Voltage"=w135, "HL.HL - DDM Parameter - Current"=w134, "HL.HL - DDM Parameter - Power"=w133, "HL.HL - DDM Parameter - Measured Power"=w131, "HL.HL - DDM Parameter - Speed"=w132, "HL.HL - DDM Parameter - Pressure"=w130, "HL_Status.HL - DDM Parameter - Voltage"=w128, "HL_Status.HL - DDM Parameter - Current"=w127, "HL_Status.HL - DDM Parameter - Power"=w126, "HL_Status.HL - DDM Parameter - Measured Power"=w125, "HL_Status.HL - DDM Parameter - Speed"=w124, "HL_Status.HL - DDM Parameter - Pressure"=w123) -> (w136:T1)
        n70 = Delete From Array(array=w147, length=1 ("长度"), index=0 ("索引")) -> (array with subset deleted=w146:bool[])  [unwired: 1 out]
        n71 = call "LogStatus.vi"("error in (no error)"=w138, "last message"=w160, "message"=w155) -> ("error  out"=w161:errorcluster)  [unwired: 8 in]
        n72 = Bundle By Name(cluster=w158, "Task_Detect_Calib.HL.DDM_Parameter"=w148, "Task_Detect_Calib.HL.DDM_Parameter_status"=w146) -> (w157:T3)
        n73 = case shown="错误" w138 {
          tunnel: [_ TRUE] -> w143
          tunnel: [_ "Error"] -> w142
          frame No Error {
          }
          frame Error {
          }
        }
      }
      frame "HL_Get_and_check_tester_Parameter" {
        n74 = Unbundle By Name(w256) -> ("Task_Detect_Calib.HL.DDM_Parameter"=w247:dbl[])
        n75 = Unbundle By Name(w244) -> ("Table"=w246:string[][], "daemon reference"=w245:refnum<k5>)
        n76 = call "Select_Table_Vaule Enable_Disable.vi"("Action"=w261, "Table"=w246) -> ("Enable"=w260:bool)  [unwired: 8 in, 1 out]
        n77 = case shown="假" w260 {
          tunnel: w245 -> [w273 w291]
          tunnel: [w273 w291] -> w242
          tunnel: [w270 w282] -> w262
          tunnel: w261 -> [_ w288]
          tunnel: w246 -> [_ w292]
          tunnel: [_ w280] -> w259
          tunnel: [_ w290] -> w251
          tunnel: w247 -> [_ w279]
          tunnel: [w271 w275] -> w243
          tunnel: [w271 w274] -> w224
          frame False {
            w270 = "Skip" ("software string")
            n78 = Initialize Array(w270, 4 ("维数大小")) -> (w271:string[])
          }
          frame True {
            w281 = string[] ["HL_Tester_Voltage", "HL_Tester_Current", "HL_Tester_Power", "HL_DDM_Real_Power"]
            n79 = call "Task_Detect_Calibration_Calculate_Tester_Parameter.vi"("DDM Parameter"=w279) -> ("Calculate Tester Parameter"=w280:dbl[])  [unwired: 10 in]
            n80 = Number To Fractional String(number=w280) -> (F-format string=w275:string[])  [unwired: 3 in]
            n81 = Interleave 1D Arrays(w281, w275) -> (w285:string[])
            n82 = Array To Spreadsheet String(delimiter (Tab)=";" ("格式字符串"), array=w285, 3:"" ("格式字符串")) -> (spreadsheet string=w282:string)
            n83 = Build Array (concatenate)(w288, w281) -> (w289:string[])
            n84 = Build Array (concatenate)("", w275) -> (w287:string[])
            n85 = for {
              tunnel: w292 -> [w298]
              tunnel: w287 -> [w296] mode=indexing
              tunnel: w289 -> [w295] mode=indexing
              tunnel: [w294] -> w290 mode=indexing
              tunnel: [w293] -> w276 mode=indexing
              w303 = "UIdisplay" ("Process (\"\" - local)")
              n86 = call "Select_Table_Vaule.vi"("Vaule"=w296, "Action"=w295, "Table"=w298) -> ("Result"=w294:bool, "vaule"=w297:string[])  [unwired: 7 in]
              n87 = Append True/False String(1:w294, 2:"FAIL" ("真字符串"), 3:"PASS" ("真字符串")) -> (0:w293:string)  [unwired: 1 in]
              n88 = Build Array (concatenate)(w297, w296, w293) -> (w302:string[])
              n89 = Flatten To XML(anything=w302) -> (xml string=w301:string)
              n90 = call "AMC Send Local Message.vi"("Process (\"\" - local)"=w303, "Message Value"=w301, "Message Name"=w303) -> ()  [unwired: 7 in, 2 out]
            }
            n91 = Delete From Array(array=w276, length=1 ("长度"), index=0 ("索引")) -> (array with subset deleted=w274:string[])  [unwired: 1 out]
          }
        }
        n92 = call <vilib>:"Space Constant.vi"() -> ("String"=w264:string)
        n93 = Concatenate Strings(w261, w264, w262) -> (w263:string)
        n94 = Unbundle By Name(w232) -> ("MES bool"=w236:refnum<vi>)
        n95 = call "HD_Config.vi"("Step"=enum16{"Initial", "Write", "Read"}."Read") -> ("HD Config out"=w237:T5)  [unwired: 9 in, 1 out]
        n96 = Unbundle By Name(w237) -> ("Fail_resume_mode"=w235:bool)
        n97 = property class="Bool (严格)"(reference=w236) -> ("Value"=w234:bool)  [unwired: 1 in, 2 out]
        n98 = Index Array(array=w243) -> (element #1=w229:string, element #2=w228:string, element #3=w227:string, element #4=w226:string)  [unwired: 4 in]
        n99 = Index Array(array=w224) -> (element #1=w225:string, element #2=w223:string, element #3=w222:string, element #4=w221:string)  [unwired: 4 in]
        n100 = Not(x=w234) -> (.not. x?=w233:bool)
        n101 = Or(x=w235, y=w233) -> (x .or. y?=w238:bool)
        n102 = Unbundle By Name(w256) -> ("Task_Detect_Calib.HL.DDM_Parameter_status"=w255:bool[])
        n103 = Delete From Array(array=w251, length=1 ("长度"), index=0 ("索引")) -> (array with subset deleted=w250:bool[])  [unwired: 1 out]
        n104 = Bundle By Name(cluster=w244, "daemon reference"=w242, "HL.HL - Tester Parameter - Voltage"=w229, "HL.HL - Tester Parameter - Current"=w228, "HL.HL - Tester Parameter - Power"=w227, "HL.HL - DDM Real Power"=w226, "HL_Status.HL - Tester Parameter - Voltage"=w225, "HL_Status.HL - Tester Parameter - Current"=w223, "HL_Status.HL - Tester Parameter - Power"=w222, "HL_Status.HL - DDM Real Power"=w221) -> (w241:T1)
        n105 = Build Array (concatenate)(w255, w250) -> (w254:bool[])
        n106 = Bundle By Name(cluster=w256, "Task_Detect_Calib.HL.Get_Tester_Parameter"=w259, "Task_Detect_Calib.HL.Get_Tester_Parameter_status"=w250) -> (w265:T3)
        n107 = call "LogStatus.vi"("error in (no error)"=w268, "last message"=w266, "message"=w263) -> ("error  out"=w267:errorcluster)  [unwired: 8 in]
        n108 = And Array Elements(Boolean array=w254) -> (logical AND=w231:bool)
        n109 = Select(t=TRUE, s=w238, f=w231) -> (s? t:f=w230:bool)
        n110 = Select(t="Calibrate_task_detect-HL(B)", s=w230, f="Finalization_NG_unit") -> (s? t:f=w252:string)
        n111 = Not(x=w230) -> (.not. x?=w253:bool)
      }
      frame "Calibrate_task_detect-HL(B)" {
        n112 = Unbundle By Name(w321) -> ("Table"=w326:string[][], "daemon reference"=w334:refnum<k5>, "Config"=w325:string[][])
        n113 = call "Select_Table_Vaule Enable_Disable.vi"("Action"=w327, "Table"=w326) -> ("Enable"=w328:bool)  [unwired: 8 in, 1 out]
        n114 = case shown="假" w328 {
          tunnel: w334 -> [w346 w364]
          tunnel: [TRUE w350] -> w307
          tunnel: [w346 w358] -> w319
          tunnel: [w345 w349] -> w329
          tunnel: w327 -> [_ w357]
          tunnel: w326 -> [_ w356]
          tunnel: w325 -> [_ _]
          tunnel: [_ w352] -> w324
          tunnel: [_ w351] -> w320
          tunnel: [_ w350] -> w322
          tunnel: [w345 w349] -> w305
          tunnel: [w345 w348] -> w304
          frame False {
            w345 = "Skip" ("response")
          }
          frame True {
            w363 = "UIdisplay" ("Process (\"\" - local)")
            n115 = call "set_task_detect.vi"("Action"=0, "Test Point"=task_detect_test_point."HL", "daemon reference in"=w364) -> ("error out"=w351:errorcluster, "response"=w349:string, "daemon reference out"=w358:refnum<k5>)  [unwired: 5 in, 1 out]
            n116 = call "Select_Table_Vaule.vi"("Vaule"=w349, "Action"=w357, "Table"=w356) -> ("Result"=w350:bool, "vaule"=w355:string[])  [unwired: 7 in]
            n117 = Fract/Exp String To Number(string=w349) -> (number=w352:dbl)  [unwired: 3 in, 1 out]
            n118 = Append True/False String(1:w350, 2:"FAIL" ("真字符串"), 3:"PASS" ("真字符串")) -> (0:w348:string)  [unwired: 1 in]
            n119 = Build Array (concatenate)(w355, w349, w348) -> (w362:string[])
            n120 = Flatten To XML(anything=w362) -> (xml string=w361:string)
            n121 = call "AMC Send Local Message.vi"("Process (\"\" - local)"=w363, "Message Value"=w361, "Message Name"=w363) -> ()  [unwired: 7 in, 2 out]
          }
        }
        n122 = call <vilib>:"Space Constant.vi"() -> ("String"=w331:string)
        n123 = Concatenate Strings(w327, w331, w329) -> (w330:string)
        n124 = Unbundle By Name(w308) -> ("MES bool"=w313:refnum<vi>)
        n125 = call "HD_Config.vi"("Step"=enum16{"Initial", "Write", "Read"}."Read") -> ("HD Config out"=w314:T5)  [unwired: 9 in, 1 out]
        n126 = Unbundle By Name(w314) -> ("Fail_resume_mode"=w312:bool)
        n127 = property class="Bool (严格)"(reference=w313) -> ("Value"=w311:bool)  [unwired: 1 in, 2 out]
        n128 = Not(x=w311) -> (.not. x?=w310:bool)
        n129 = Bundle By Name(cluster=w321, "HL_Status.HL - Calibrate Task Detect HL"=w304, "HL.HL - Calibrate Task Detect HL"=w305, "daemon reference"=w319) -> (w318:T1)
        n130 = Or(x=w312, y=w310) -> (x .or. y?=w315:bool)
        n131 = Select(t=TRUE, s=w315, f=w307) -> (s? t:f=w306:bool)
        n132 = Bundle By Name(cluster=w333, "Task_Detect_Calib.HL.Set_task_detect_B"=w324, "Task_Detect_Calib.HL.Set_task_detect_B_Status"=w322) -> (w332:T3)
        n133 = case shown="无错误" w320 {
          tunnel: [w339 TRUE] -> w323
          tunnel: [w341 "Error"] -> w317
          tunnel: w306 -> [w338 _]
          frame No Error {
            n134 = Select(t="HL_Motor_Stop", s=w338, f="Finalization_NG_unit") -> (s? t:f=w341:string)
            n135 = Not(x=w338) -> (.not. x?=w339:bool)
          }
          frame Error {
          }
        }
        n136 = call "LogStatus.vi"("error in (no error)"=w320, "last message"=w335, "message"=w330) -> ("error  out"=w336:errorcluster)  [unwired: 8 in]
      }
      frame "HL_Motor_Stop" {
        n137 = Unbundle By Name(w368) -> ("Table"=w374:string[][], "daemon reference"=w379:refnum<k5>, "Config"=w373:string[][])
        n138 = call "Select_Table_Vaule Enable_Disable.vi"("Action"=w375, "Table"=w374) -> ("Enable"=w376:bool)  [unwired: 8 in, 1 out]
        n139 = case shown="真" w376 {
          tunnel: w379 -> [w386 w402]
          tunnel: [TRUE w392] -> _
          tunnel: [w386 w396] -> w365
          tunnel: ["" ("response") w391] -> w370
          tunnel: w375 -> [_ w395]
          tunnel: w374 -> [_ w394]
          tunnel: w373 -> [_ _]
          tunnel: [_ w388] -> w366
          tunnel: [_ w391] -> _
          tunnel: [_ w390] -> _
          tunnel: [_ w389] -> _
          frame False {
          }
          frame True {
            w389 = "STOP" ("Power Mode")
            w401 = "UIdisplay" ("Process (\"\" - local)")
            n140 = call "drive_motor.vi"("Power Mode"=w389, "daemon reference in"=w402) -> ("error out"=w388:errorcluster, "response"=w391:string, "daemon reference out"=w396:refnum<k5>)  [unwired: 6 in, 1 out]
            n141 = call "时间延迟"("error in (no error)"=w388) -> ()  [unwired: 10 in, 1 out]
            n142 = call "Select_Table_Vaule.vi"("Vaule"=w391, "Action"=w395, "Table"=w394) -> ("Result"=w392:bool, "vaule"=w393:string[])  [unwired: 7 in]
            n143 = Append True/False String(1:w392, 2:"FAIL" ("真字符串"), 3:"PASS" ("真字符串")) -> (0:w390:string)  [unwired: 1 in]
            n144 = Build Array (concatenate)(w393, w391, w390) -> (w400:string[])
            n145 = Flatten To XML(anything=w400) -> (xml string=w399:string)
            n146 = call "AMC Send Local Message.vi"("Process (\"\" - local)"=w401, "Message Value"=w399, "Message Name"=w401) -> ()  [unwired: 7 in, 2 out]
          }
        }
        n147 = call <vilib>:"Space Constant.vi"() -> ("String"=w378:string)
        n148 = Concatenate Strings(w375, w378, w370) -> (w377:string)
        n149 = Bundle By Name(cluster=w368, "daemon reference"=w365) -> (w367:T1)
        n150 = call "LogStatus.vi"("error in (no error)"=w366, "last message"=w380, "message"=w377) -> ("error  out"=w381:errorcluster)  [unwired: 8 in]
        n151 = case shown="错误" w366 {
          tunnel: ["LH_Restriction" "Error"] -> w371
          frame No Error {
          }
          frame Error {
          }
        }
      }
    }
    n152 = call "6-AlarmStatus.vi"("Step"=enum16{"Initial", "Write", "Read"}."Read") -> ("AlarmValue Out"=w18:bool[])  [unwired: 9 in, 1 out]
    n153 = call "Stop.vi"("Step"=enum16{"Initial", "Write", "Read"}."Read") -> ("Stop Out"=w26:bool)  [unwired: 9 in, 1 out]
    n154 = call "Exit.vi"("Step"=enum16{"Initial", "Write", "Read"}."Read" ("step")) -> ("Exit Out"=w25:bool)  [unwired: 9 in, 1 out]
    n155 = Or Array Elements(Boolean array=w18) -> (logical OR=w17:bool)
    n156 = Compound Arithmetic op=OR(w24, w26, w25, w17) -> (w23:bool)
    n157 = call "AMC Run Step.vi"("Message Queue In"=w44, "Message Name"=w32, "Message Value"=w30, "error in (no error)"=w39, "Mli/Sig"=FALSE) -> ("Message Queue Out"=w43:T4, "error out"=w38:errorcluster)  [unwired: 13 in]
  }
  "Message Queue Out" <- w6
  "error out" <- w5
  "Data" <- w10
  "Flow" <- w7
  "Data out" <- w1
